vi "Generate GUID.vi"(8 "error in (no error)":errorcluster) -> (0 "error out":errorcluster, 3 "New GUID":string)   [LabVIEW 2020, in "ADAS_IO_Template_MDO.lvclass"]
uses:
  ADAS_IO_Template_MDO.lvclass
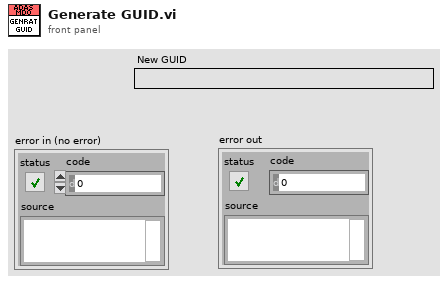
[diagram p1: front panel]
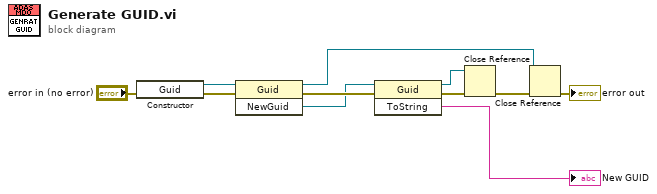
[diagram p0: block diagram]
diagram:
  n1 = constructor class="Guid"(error in="error in (no error)") -> (reference out=w10:refnum<k24>, error out=w11:errorcluster)  [unwired: 2 in, 1 out]
  n2 = invoke class="Guid" method="NewGuid"(reference=w10, error in=w11) -> (reference out=w3:refnum<k24>, error out=w9:errorcluster, "NewGuid"=w8:refnum<k24>)  [unwired: 1 in]
  n3 = invoke class="Guid" method="ToString"(reference=w8, error in=w9) -> (reference out=w4:refnum<k24>, error out=w6:errorcluster, "ToString"=→"New GUID":string)  [unwired: 1 in]
  n4 = Close Reference(reference=w4, error in (no error)=w6) -> (error out=w5:errorcluster)
  n5 = Close Reference(reference=w3, error in (no error)=w5) -> (error out=→"error out":errorcluster)
